vi "CIMAQ_Cast_Binary_RGB.vi"(8 "error in":errorcluster, 10 "Dest (optional)":T1=refnum, 11 "Source":T1) -> (0 "error out":errorcluster, 3 "Result":T1)   [LabVIEW 2017]
uses:
  <vilib>/vision/Image Controls.llb/IMAQ Image.ctl
  <vilib>/vision/NI_Vision_Development_Module.lvlib
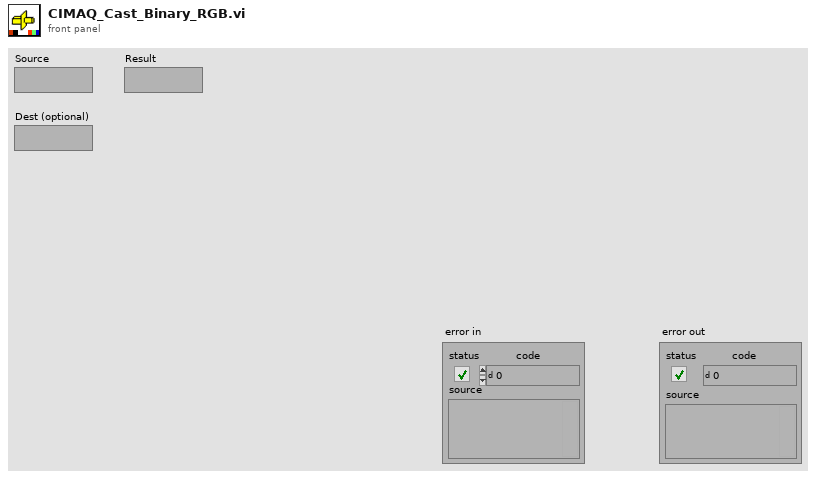
[diagram p1: front panel]
types:
  T1 = typedef "IMAQ Image.ctl" = refnum<image>
  T2 = typedef "Image Type" = u32
  T3 = enum32{"Gray", "Binary", "Gradient", "Rainbow", "Temperature"}
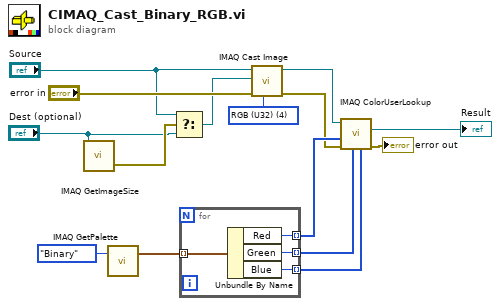
[diagram p0: block diagram]
diagram:
  w1 = T2 4 items=["Grayscale (U8)", "Grayscale (I16)", "Grayscale (SGL)", "Complex (CSG)", "RGB (U32)", "HSL (U32)", "RGB (U64)", "Grayscale (U16)"] ("Image Type")
  n1 = call "IMAQ GetImageSize"("Image"="Dest (optional)") -> ("error out"=w5:errorcluster)  [unwired: 3 in, 2 out]
  n2 = call "IMAQ GetPalette"("Palette Number (gray)"=T3."Binary") -> ("Color Palette"=w11:cluster{"Red":u8, "Green":u8, "Blue":u8}[])  [unwired: 4 in, 1 out]
  n3 = Select(t="Source", s=w5, f="Dest (optional)") -> (s? t:f=w2:T1)
  n4 = for {
    tunnel: w11 -> [w19] mode=indexing
    tunnel: [w18] -> w14 mode=indexing
    tunnel: [w17] -> w13 mode=indexing
    tunnel: [w16] -> w12 mode=indexing
    n5 = Unbundle By Name(w19) -> ("Red"=w16:u8, "Green"=w17:u8, "Blue"=w18:u8)
  }
  n6 = call "IMAQ Cast Image"("Image Type"=w1, "error in (no error)"="error in", "Image Dst"=w2, "Image Src"="Source") -> ("error out"=w7:errorcluster, "Image Dst Out"=w6:T1)  [unwired: 6 in]
  n7 = call "IMAQ ColorUserLookup"("Blue or Luma or Val or Inten Lookup Table"=w14, "Green or Sat Lookup Table"=w13, "error in (no error)"=w7, "Red or Hue Lookup Table"=w12, "Image Src"=w6) -> ("error out"=→"error out":errorcluster, "Image Dst Out"=→"Result":T1)  [unwired: 5 in]
